vi "Hulling_Process (SubVI).vi"(10 "Array in":string[](array[string]), 11 "Digital in":refnum<vi>) -> (1 "Array out":string[](array[string]), 2 "Boolean":bool, 3 "empty?":bool)   [LabVIEW 2019]
uses:
  <vilib>/numeric/Random Number (Range) DBL.vi
  68a865dd-50af-4b5d-a3bf-14e6e21a10e7.vi
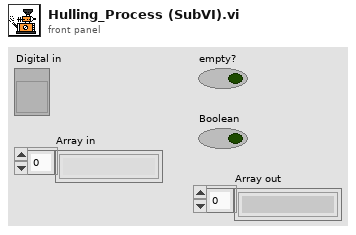
[diagram p1: front panel]
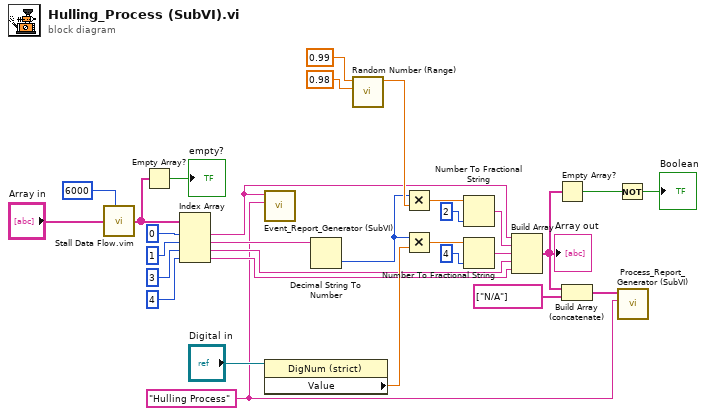
[diagram p0: block diagram]
diagram:
  w1 = "Hulling Process" ("Process Name")
  n1 = call "Stall Data Flow.vim"("value in"="Array in", "milliseconds to wait"=u32 6000) -> ("value out"=w8:string[])  [unwired: 1 out]
  n2 = Empty Array?(array=w8) -> (empty?=→"empty?":bool)
  n3 = Index Array(array=w8, index #1=0 ("index"), index #2=1 ("index"), index #3=3 ("index"), index #4=4 ("index")) -> (element #1=w5:string, element #2=w23:string, element #3=w20:string, element #4=w19:string)
  n4 = call "Event_Report_Generator (SubVI).vi"("Process Name"=w1, "Booking ID"=w5) -> ()  [unwired: 10 in]
  n5 = property class="DigNum (strict)"(reference="Digital in") -> ("Value"=w26:dbl)  [unwired: 1 in, 2 out]
  n6 = Decimal String To Number(string=w23) -> (number=w21:i32)  [unwired: 2 in, 1 out]
  n7 = call-poly <vilib>:"Random Number (Range).vi"("lower bound (0)"=0.98, "upper bound (100)"=0.99) -> ("number"=w22:dbl)  [unwired: 9 in]
  n8 = Multiply(x=w21, y=w22) -> (x*y=w24:dbl)
  n9 = Multiply(x=w21, y=w26) -> (x*y=w25:dbl)
  n10 = Number To Fractional String(number=w24, precision (6)=i16 2) -> (F-format string=w28:string)  [unwired: 2 in]
  n11 = Number To Fractional String(number=w25, precision (6)=i16 4) -> (F-format string=w27:string)  [unwired: 2 in]
  n12 = Build Array(w5, w28, w27, w20, w19) -> (w4:string[])
  "Array out" <- w4
  n13 = Empty Array?(array=w4) -> (empty?=w29:bool)
  n14 = Build Array (concatenate)(w4, string[] ["N/A"] ("array")) -> (w2:string[])
  n15 = Not(x=w29) -> (.not. x?=→"Boolean":bool)
  n16 = call "Process_Report_Generator (SubVI).vi"("Process Name"=w1, "Process Information"=w2) -> ()  [unwired: 10 in]
